vi "CloseSocketListener.vi"(0 "Universal Robot.lvclass in":refnum<class "Universal Robot.lvclass">, 5 "Error In":errorcluster) -> (14 "Universal Robot.lvclass out":refnum<class "Universal Robot.lvclass">)   [LabVIEW 2019, in "Universal Robot.lvclass"]
uses:
  Universal Robot.lvclass
  Universal Robot.lvclass/Universal Robot.ctl
  Client Interfaces/Socket Communication/Socket Communication.lvclass
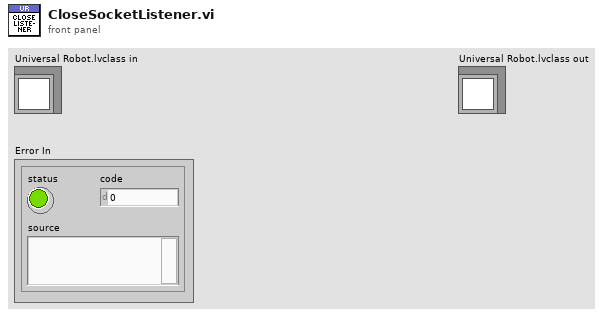
[diagram p1: front panel]
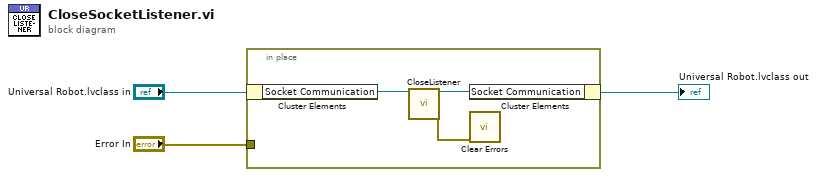
[diagram p0: block diagram]
diagram:
  n1 = in-place {
    in-place-border: "Error In" -> [_]
    n2 = in-place-cluster #1("Universal Robot.lvclass in") -> ("Socket Communication"=w6:refnum<class "Socket Communication.lvclass">)
    n3 = call-dynamic "CloseListener.vi"("TCP Socket in"=w6) -> ("TCP Socket out"=w5:refnum<class "Socket Communication.lvclass">, "error out"=w4:errorcluster)  [unwired: 17 in]
    n4 = in-place-cluster #1("Socket Communication"=w5) -> (→"Universal Robot.lvclass out":refnum<class "Universal Robot.lvclass">)
    n5 = call <vilib>:"Clear Errors.vi"("error in (no error)"=w4) -> ()  [unwired: 5 in, 2 out]
  }
